vi "SignalOutputV3.vi"(1 "signal cluster 2":T1, 2 "Gain Type":string, 3 "SetInstrument Cluster":cluster{dbl, dbl, dbl, dbl[], dbl, dbl, dbl}) -> (0 "Signal output":dbl)   [LabVIEW 2011]
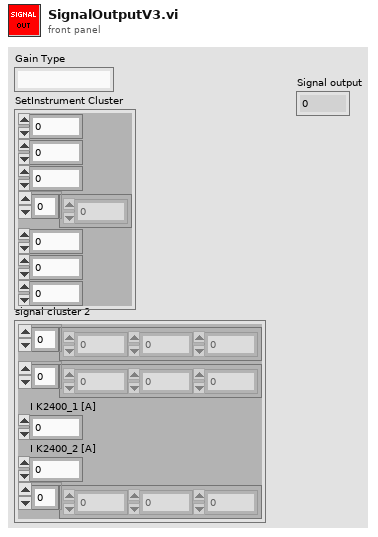
[diagram p1: front panel]
types:
  T1 = cluster{dbl[], dbl[], "I K2400_1 [A]":dbl, "I K2400_2 [A]":dbl, dbl[]}
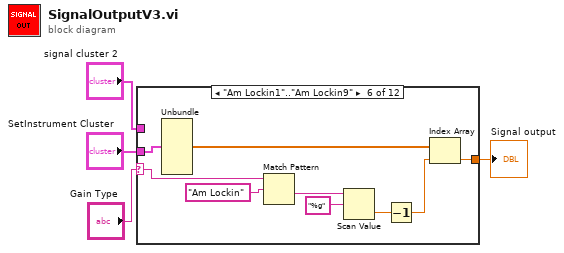
[diagram p0: block diagram]
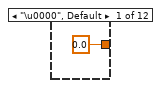
[diagram p2: hidden frame]
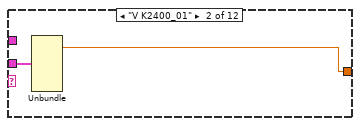
[diagram p3: hidden frame]
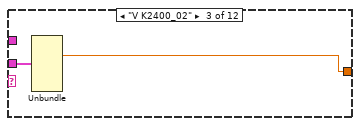
[diagram p4: hidden frame]
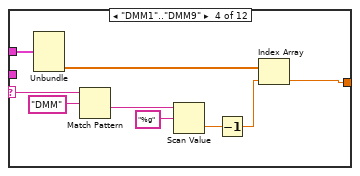
[diagram p5: hidden frame]
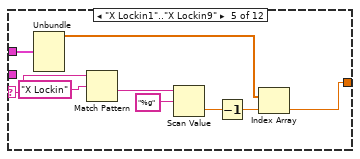
[diagram p6: hidden frame]
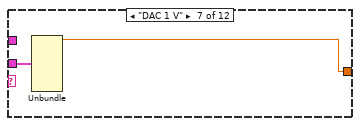
[diagram p7: hidden frame]
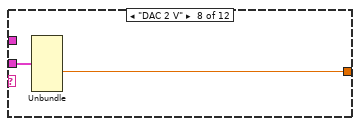
[diagram p8: hidden frame]
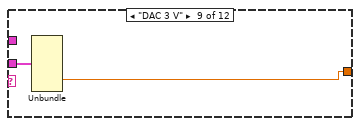
[diagram p9: hidden frame]
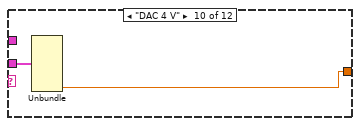
[diagram p10: hidden frame]
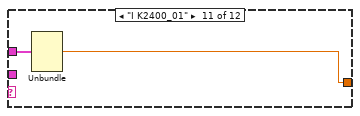
[diagram p11: hidden frame]
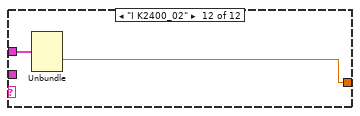
[diagram p12: hidden frame]
diagram:
  n1 = case shown="\"Am Lockin1\"..\"Am Lockin9\"" "Gain Type" {
    selector: "Gain Type" -> [_ _ _ w14 w23 w33 _ _ _ _ _ _]
    tunnel: "SetInstrument Cluster" -> [_ w7 w9 _ _ w29 w38 w40 w42 w44 _ _]
    tunnel: "signal cluster 2" -> [_ _ _ w18 w27 _ _ _ _ _ w46 w48]
    tunnel: [0.0 ("I K2400_2 [A]") w6 w8 w11 w21 w31 w37 w39 w41 w43 w45 w47] -> w3
    frame "\u0000", Default {
    }
    frame "V K2400_01" {
      n2 = Unbundle(w7) -> (w6:dbl)  [unwired: 6 out]
    }
    frame "V K2400_02" {
      n3 = Unbundle(w9) -> (w8:dbl)  [unwired: 6 out]
    }
    frame "DMM1".."DMM9" {
      n4 = Unbundle(w18) -> (w13:dbl[])  [unwired: 4 out]
      n5 = Match Pattern(string=w14, regular expression="DMM") -> (after substring=w16:string)  [unwired: 1 in, 3 out]
      n6 = Scan Value(string=w16, format string="%g") -> (value=w12:dbl)  [unwired: 1 in, 1 out]
      n7 = Decrement(x=w12) -> (x-1=w10:dbl)
      n8 = Index Array(array=w13, index=w10) -> (element=w11:dbl)
    }
    frame "X Lockin1".."X Lockin9" {
      n9 = Unbundle(w27) -> (w19:dbl[])  [unwired: 4 out]
      n10 = Match Pattern(string=w23, regular expression="X Lockin") -> (after substring=w25:string)  [unwired: 1 in, 3 out]
      n11 = Scan Value(string=w25, format string="%g") -> (value=w22:dbl)  [unwired: 1 in, 1 out]
      n12 = Decrement(x=w22) -> (x-1=w20:dbl)
      n13 = Index Array(array=w19, index=w20) -> (element=w21:dbl)
    }
    frame "Am Lockin1".."Am Lockin9" {
      n14 = Unbundle(w29) -> (w28:dbl[])  [unwired: 6 out]
      n15 = Match Pattern(string=w33, regular expression="Am Lockin") -> (after substring=w35:string)  [unwired: 1 in, 3 out]
      n16 = Scan Value(string=w35, format string="%g") -> (value=w32:dbl)  [unwired: 1 in, 1 out]
      n17 = Decrement(x=w32) -> (x-1=w30:dbl)
      n18 = Index Array(array=w28, index=w30) -> (element=w31:dbl)
    }
    frame "DAC 1 V" {
      n19 = Unbundle(w38) -> (w37:dbl)  [unwired: 6 out]
    }
    frame "DAC 2 V" {
      n20 = Unbundle(w40) -> (w39:dbl)  [unwired: 6 out]
    }
    frame "DAC 3 V" {
      n21 = Unbundle(w42) -> (w41:dbl)  [unwired: 6 out]
    }
    frame "DAC 4 V" {
      n22 = Unbundle(w44) -> (w43:dbl)  [unwired: 6 out]
    }
    frame "I K2400_01" {
      n23 = Unbundle(w46) -> ("I K2400_1 [A]"=w45:dbl)  [unwired: 4 out]
    }
    frame "I K2400_02" {
      n24 = Unbundle(w48) -> ("I K2400_2 [A]"=w47:dbl)  [unwired: 4 out]
    }
  }
  "Signal output" <- w3
